vi "ActualizarTablaFrecuencia.vi"(8 "error in (no error)":errorcluster, 10 "medido":dbl, 11 "Prueba21_1":refnum<class "Prueba21.lvclass">) -> (0 "error out":errorcluster, 3 "Prueba21_1":refnum<class "Prueba21.lvclass">)   [LabVIEW 2019, in "Prueba21.lvclass"]
uses:
  Prueba21.lvclass
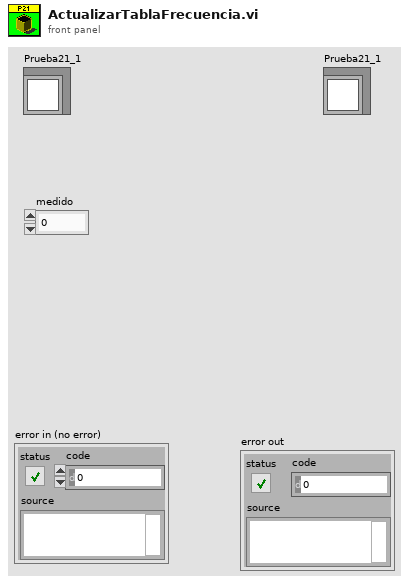
[diagram p1: front panel]
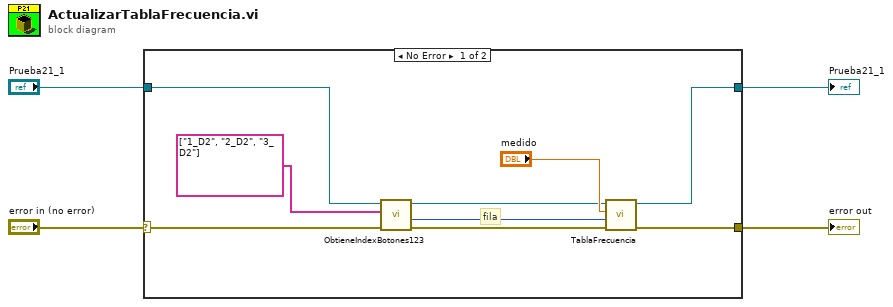
[diagram p0: block diagram]
diagram:
  n1 = case shown="No Error" "error in (no error)" {
    selector: "error in (no error)" -> [w8 w14]
    tunnel: [w13 w15] -> w4
    tunnel: [w11 w14] -> w3
    tunnel: "Prueba21_1" -> [w10 w15]
    frame No Error {
      # "fila"
      n2 = call "ObtieneIndexBotones123.vi"("error in (no error)"=w8, "Botones"=string[] ["1_D2", "2_D2", "3_D2"], "Prueba21_1 in"=w10) -> ("error out"=w9:errorcluster, "index of element"=w6:i32, "Prueba21_1 out"=w7:refnum<class "Prueba21.lvclass">)  [unwired: 6 in]
      n3 = call "TablaFrecuencia.vi"("error in (no error)"=w9, "fila"=w6, "FrecuenciaMedida"="medido", "Prueba21_1 in"=w7) -> ("error out"=w11:errorcluster, "Prueba21_1 out"=w13:refnum<class "Prueba21.lvclass">)  [unwired: 6 in]
    }
    frame Error {
    }
  }
  "Prueba21_1" <- w4
  "error out" <- w3
